vi "Handle Last Ack Core.vi"(4 "error in (no error)":errorcluster, 6 "Last Ack":refnum<class "Last Ack.lvclass">, 7 "Process Model in":refnum<class "Process Model.lvclass">) -> (0 "error out":errorcluster, 3 "Process Model out":refnum<class "Process Model.lvclass">)   [LabVIEW 2019, in "Process Model.lvclass"]
doc: "(<B>Filename</B>: Actor Framework.lvlib:Actor.lvclass:Handle Last Ack Core.vi)\n\nDefines how the caller actor responds to the Last Ack message from a nested actor. The Last Ack message is the final message a nested actor sends to its caller before it shuts down. The message contains information about the final state of the nested actor.\n\nBy default, this method does nothing except return any error the nested actor sent. A descendant class may override this method to define behavior."
uses:
  <vilib>/gpm_packages/@cs/Car-wash/Source/Process Model/Process Model.lvclass
  <vilib>/ActorFramework/LastAck/Last Ack.lvclass
  C:/Program Files/National Instruments/LabVIEW 2019/vi.lib/ActorFramework/Actor/Actor.lvclass
  <vilib>/ActorFramework/LastAck/Last Ack.lvclass/Last Ack.ctl
  <vilib>/gpm_packages/@cs/Car-wash/Source/iProcess Step Model/iProcess Step Model/iProcess Step Model.lvclass
  <vilib>/gpm_packages/@cs/Car-wash/Source/Process Model/Process Model.lvclass/Process Model.ctl
  <vilib>/ActorFramework/Actor/Actor.lvclass/Actor.ctl
  <vilib>/ActorFramework/Message Enqueuer/Message Enqueuer.lvclass/Message Enqueuer.ctl
  <vilib>/ActorFramework/Message Enqueuer/Message Enqueuer.lvclass
  <vilib>/ActorFramework/Message Enqueuer/Init from Existing Queue.vi
  <vilib>/ActorFramework/Message Enqueuer/Enqueue.vi
  <vilib>/gpm_packages/@cs/Car-wash/Source/iProcess Model/iProcess Model Messages/Execute Process Msg/Execute Process Step Msg.lvclass
  C:/Program Files/National Instruments/LabVIEW 2019/vi.lib/ActorFramework/Message/Message.lvclass
  <vilib>/ActorFramework/Message Priority Queue/Priority Enqueue.vi
  <vilib>/gpm_packages/@cs/Car-wash/Source/iProcess Model/iProcess Model/iProcess Model.lvclass
  <vilib>/ActorFramework/Actor/Actor.lvclass
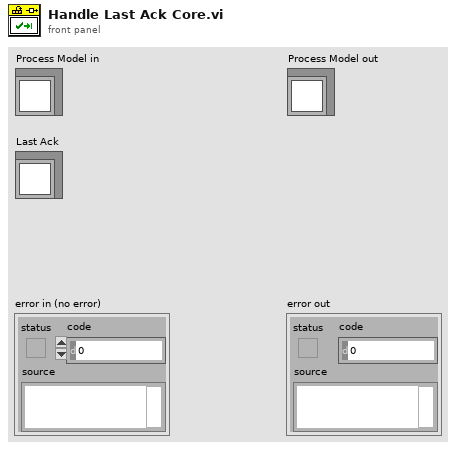
[diagram p1: front panel]
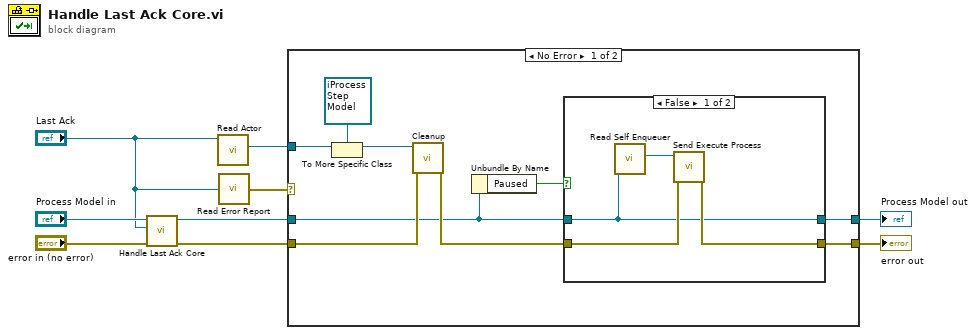
[diagram p0: block diagram]
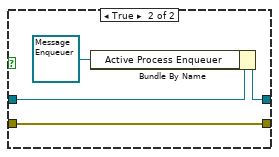
[diagram p2: hidden frame]
diagram:
  n1 = call-parent "Handle Last Ack Core.vi"("error in (no error)"="error in (no error)", "Last Ack"="Last Ack", "IModel in"="Process Model in") -> ("error out"=w5:errorcluster, "IModel out"=w3:refnum<class "Process Model.lvclass">)  [unwired: 3 in]
  n2 = call <vilib>:"Read Actor.vi"("Last Ack"="Last Ack") -> ("Actor"=w6:refnum<class "Actor.lvclass">)  [unwired: 10 in]
  n3 = call <vilib>:"Read Error Report.vi"("Last Ack"="Last Ack") -> ("error report"=w1:errorcluster)
  n4 = case shown="No Error" w1 {
    selector: w1 -> [_ w27]
    tunnel: w6 -> [w18 _]
    tunnel: w5 -> [w15 _]
    tunnel: [w13 w27] -> w4
    tunnel: w3 -> [w12 w28]
    tunnel: [w11 w28] -> w2
    frame No Error {
      n5 = To More Specific Class(target class=refnum<class "iProcess Step Model.lvclass"> refnum ("iProcess Step Model.lvclass"), reference=w18) -> (specific class reference=w16:refnum<class "iProcess Step Model.lvclass">)  [unwired: 1 in, 1 out]
      n6 = call-dynamic "Cleanup.vi"("error in (no error)"=w15, "iProcess Step Model in"=w16) -> ("error out"=w14:errorcluster)  [unwired: 8 in, 1 out]
      n7 = Unbundle By Name(w12) -> ("Paused"=w10:bool)
      n8 = case shown="False" w10 {
        tunnel: w14 -> [w21 w26]
        tunnel: [w20 w26] -> w13
        tunnel: w12 -> [w19 w25]
        tunnel: [w19 w24] -> w11
        frame False {
          n9 = call <vilib>:"Read Self Enqueuer.vi"("Actor"=w19) -> ("Self Enqueuer"=w22:refnum<class "Message Enqueuer.lvclass">)  [unwired: 10 in]
          n10 = call <vilib>:"Send Execute Process.vi"("error in (no error)"=w21, "Message Enqueuer"=w22) -> ("error out"=w20:errorcluster)  [unwired: 8 in, 1 out]
        }
        frame True {
          n11 = Bundle By Name(cluster=w25, "Active Process Enqueuer"=refnum<class "Message Enqueuer.lvclass"> refnum) -> (w24:refnum<class "Process Model.lvclass">)
        }
      }
    }
    frame Error {
    }
  }
  "Process Model out" <- w2
  "error out" <- w4
